vi "Tell Child.vi"(4 "Priority":bool, 6 "UID":string, 7 "Actor in":refnum<class "Actor.lvclass">) -> (0 "Error out":errorcluster)   [LabVIEW 2025, in "jettl.lvlib" / "Stop Msg.lvlib"]
uses:
  Stop Msg.lvlib
  Stop Msg/Stop Msg.lvclass
  C:/git/jettl/src/jettl/jettl/Stop Msg/Destroy Msg/Stop Msg.lvclass
  C:/git/jettl/src/jettl/jettl/Msg/Msg.lvclass
  Actor/Actor/Actor.lvclass
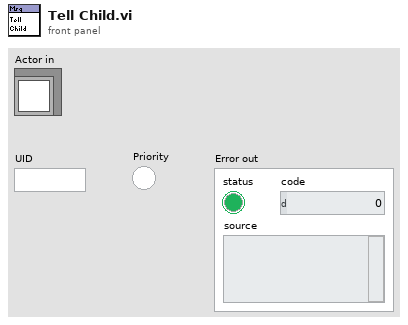
[diagram p1: front panel]
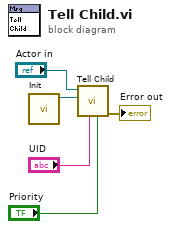
[diagram p0: block diagram]
diagram:
  n1 = call "Init.vi"() -> ("Stop Msg out"=w1:refnum<class "Stop Msg.lvclass">)  [unwired: 11 in]
  n2 = call-dynamic "Tell Child.vi"("Priority"="Priority", "UID"="UID", "Msg"=w1, "Actor in"="Actor in") -> ("Error out"=→"Error out":errorcluster)  [unwired: 7 in]
